vi "readData_NEW-SD.vi"(0 "number of aq":i32) -> (1 "I channel seq":T1, 2 "II channel seq":T1)   [LabVIEW 2015]
uses:
  controls/data-cluster.ctl
  globalVarSD.vi
panel:
  out "time of aq NEW":u32
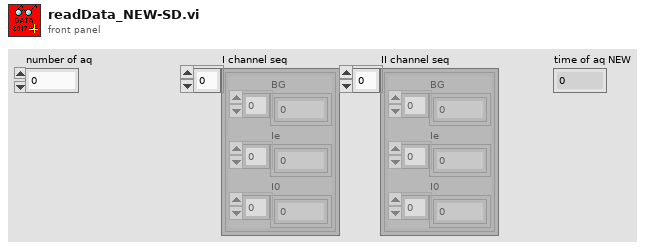
[diagram p1: front panel]
types:
  T1 = typedef "data-cluster.ctl" = cluster{"BG":i32[], "Ie":i32[], "I0":i32[]}[]
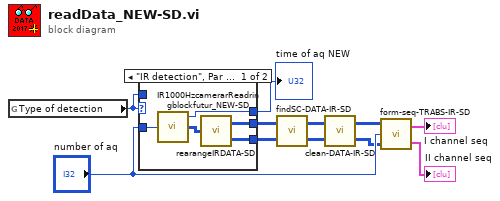
[diagram p0: block diagram]
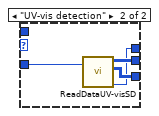
[diagram p2: hidden frame]
diagram:
  n1 = global read "globalVarSD.vi" "Type of detection"() -> (w3:enum32{"IR detection", "UV-vis detection"})
  n2 = case shown="\"IR detection\", Par défaut" w3 {
    tunnel: [w16 w18] -> w10
    tunnel: "number of aq" -> [w15 w17]
    tunnel: w3 -> [_ _]
    tunnel: [w13 w20] -> w2
    tunnel: [w12 w19] -> w1
    frame "IR detection", Default {
      n3 = call "IR1000HzcamerarReadringblockfutur_NEW-SD.vi"("Nombre d'acquisitions"=w15) -> ("temps d'acqu ms"=w16:u32, "Data THz1000Hz"=w14:u32[][])  [unwired: 1 out]
      n4 = call "rearangeIRDATA-SD.vi"("Brut camera"=w14) -> ("I channel"=w13:u16[][], "II channel"=w12:u16[][])
    }
    frame "UV-vis detection" {
      n5 = call "ReadDataUV-visSD.vi"("Nombre de aq"=w17) -> ("Channel I"=w20:i32[][], "Channel II"=w19:i32[][], "temps d'acqu ms"=w18:u32)  [unwired: 1 in, 1 out]
    }
  }
  "time of aq NEW" <- w10
  n6 = call "findSC-DATA-IR-SD.vi"("II channel"=w1, "I channel"=w2) -> ("II channel"=w5:u16[][], "I channel"=w6:u16[][])
  n7 = call "clean-DATA-IR-SD.vi"("II channel"=w5, "I channel"=w6) -> ("II channel cleaned"=w7:u16[][], "I channel cleaned"=w8:u16[][])
  n8 = call "form-seq-TRABS-IR-SD.vi"("II channel"=w7, "Number of aq"="number of aq", "I channel"=w8) -> ("II channel seq"=→"II channel seq":cluster{"BG":i32[], "Ie":u32[], "I0":i32[]}[], "I channel seq"=→"I channel seq":cluster{"BG":i32[], "Ie":i32[], "I0":i32[]}[])
